vi "WM Input Settings.vi"(1 "Input Settings":T1={"Input Device"=1, "Input Channel"="0", "Input Offset"=0.0, "Input Calibration"=1.0} {"Input Calibration" format="%.4f"; "Input Offset" format="%.4f"}) -> (0 "Input Settings Out":T1={"Input Device"=1, "Input Channel"="0", "Input Offset"=0.0, "Input Calibration"=0.0} {"Input Calibration" format="%.2f"; "Input Offset" format="%.2f"})   [LabVIEW 2012]
panel:
  in  "OK":bool
  # "V"
  # "m/V"
  # "V"
  # "m/V"
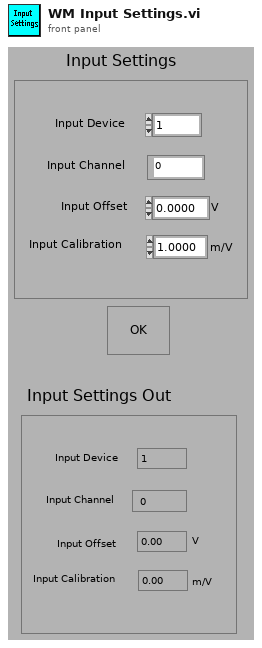
[diagram p1: front panel]
types:
  T1 = cluster{"Input Device":i32, "Input Channel":string, "Input Offset":dbl, "Input Calibration":dbl}
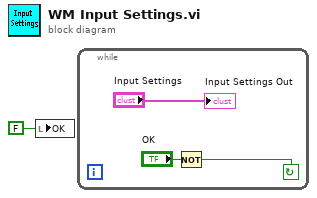
[diagram p0: block diagram]
diagram:
  n1 = local write "OK"(FALSE ("OK")) -> ()
  n2 = while {
    stop <- w3 continue-if-true
    n3 = Not(x="OK") -> (.not. x?=w3:bool)
    "Input Settings Out" <- "Input Settings"
  }
